vi "MTMount_getNextSample_CameraCableWrap.vi"(8 "error in (no error)":errorcluster, 11 "Camera_Cable_Wrap_Ctl":T1) -> (0 "error out":errorcluster, 2 "function return":i32, 3 "Camera_Cable_Wrap_Ctl out":T1)   [LabVIEW 2018, in "SALLV_MTMount.lvlib"]
doc: "int MTMount_shm_getNextSample_Camera_Cable_WrapLV(MTMount_Camera_Cable_WrapLV *Camera_Cable_Wrap_Ctl );"
uses:
  SALLV_MTMount.lvlib
  DataTypes/Camera_Cable_Wrap.ctl
  SALLV_MTMount.so
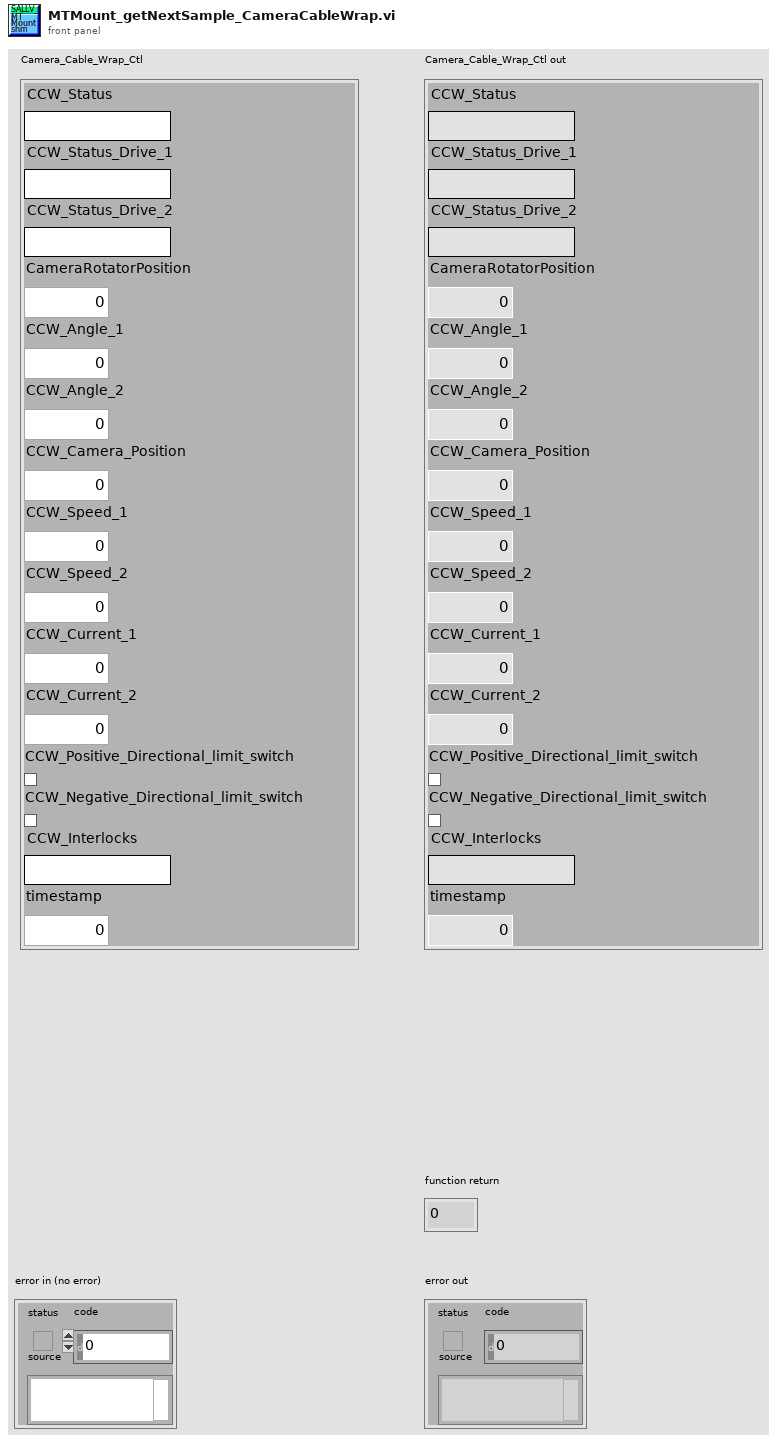
[diagram p1: front panel]
types:
  T1 = typedef "SALLV_MTMount.lvlib/Camera_Cable_Wrap.ctl" = cluster{"CCW_Status":string, "CCW_Status_Drive_1":string, "CCW_Status_Drive_2":string, "CameraRotatorPosition":dbl, "CCW_Angle_1":dbl, "CCW_Angle_2":dbl, "CCW_Camera_Position":dbl, "CCW_Speed_1":dbl, "CCW_Speed_2":dbl, "CCW_Current_1":dbl, "CCW_Current_2":dbl, "CCW_Positive_Directional_limit_switch":bool, "CCW_Negative_Directional_limit_switch":bool, "CCW_Interlocks":string, "timestamp":dbl}
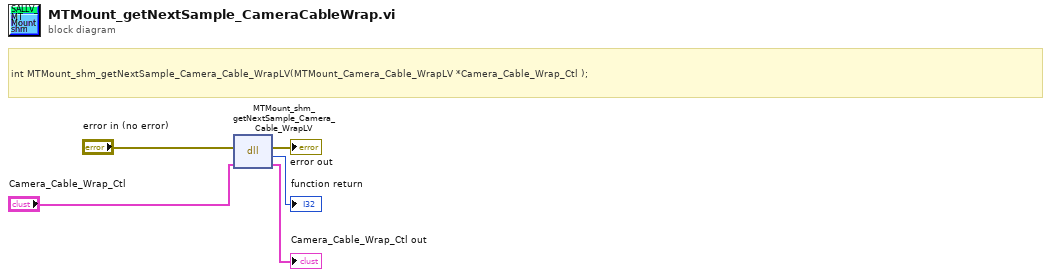
[diagram p0: block diagram]
diagram:
  # "int MTMount_shm_getNextSample_Camera_Cable_WrapLV(MTMount_Camera_Cable_WrapLV *Camera_Cable_Wrap_Ctl );"
  n1 = dll-call lib="home/ttsai/Document/salApiMTMount/SALLV_MTMount/SALLV_MTMount.*" fn="MTMount_shm_getNextSample_Camera_Cable_WrapLV"(error in="error in (no error)", "Camera_Cable_Wrap_Ctl"="Camera_Cable_Wrap_Ctl") -> (error out=→"error out":errorcluster, →"function return":i32, "Camera_Cable_Wrap_Ctl"=→"Camera_Cable_Wrap_Ctl out":T1)  [unwired: 2 in, 1 out]
